vi "SetParam.vi"(8 "error in (no error)":errorcluster caption="entrée d'erreur (pas d'erreur)", 10 "make_friedman1":T1={"n_samples"=100, "n_features"=10, "noise"=0.0, "random_state"=-1, "Returns"="X"} {"n_features" min=5; "n_samples" min=1}, 11 "Friedman1.lvclass":refnum<class "Friedman1.lvclass">) -> (0 "error out":errorcluster caption="sortie d'erreur", 3 "Friedman1.lvclass":refnum<class "Friedman1.lvclass">)   [LabVIEW 2020, in "Friedman1.lvclass"]
doc: "Set Parameters"
uses:
  Friedman1.lvclass
  Friedman1.lvclass/Friedman1.ctl
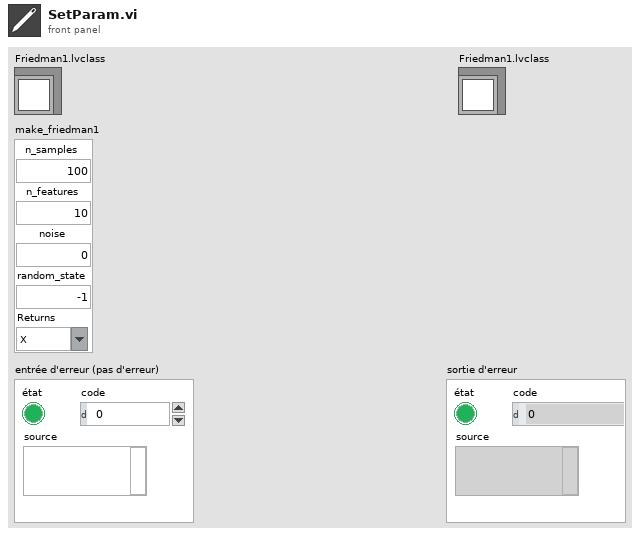
[diagram p1: front panel]
types:
  T1 = cluster{"n_samples":u32, "n_features":u32, "noise":dbl, "random_state":i32, "Returns":string}
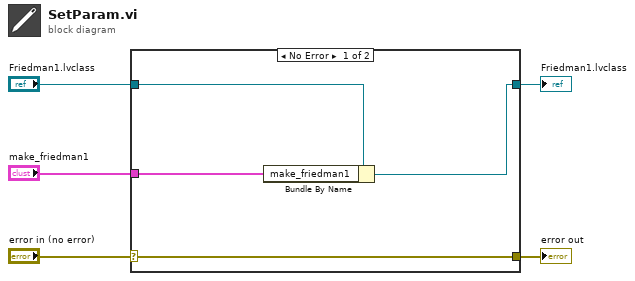
[diagram p0: block diagram]
diagram:
  n1 = case shown="No Error" "error in (no error)" {
    selector: "error in (no error)" -> [w9 w10]
    tunnel: [w9 w10] -> w4
    tunnel: [w7 w11] -> w2
    tunnel: "Friedman1.lvclass" -> [w8 w11]
    tunnel: "make_friedman1" -> [w6 _]
    frame No Error {
      n2 = Bundle By Name(cluster=w8, "make_friedman1"=w6) -> (w7:refnum<class "Friedman1.lvclass">)
    }
    frame Error {
    }
  }
  "error out" <- w4
  "Friedman1.lvclass" <- w2
